vi "Driveshift.vi"(7 "GO BUTTON":bool, 10 "Shift down override":bool, 11 "Shift up override":bool) -> ()   [LabVIEW 2013]
uses:
  <vilib>/Rock Robotics/WPI/Solenoid/WPI_SolenoidValue.ctl
  Robot Global Data.vi
  <vilib>/Rock Robotics/WPI/Solenoid/WPI_SolenoidSetEnum.vi
panel:
  out "Solenoid Value":T1
  in  "Shift Speed":dbl=4.5
  in  "Value":bool
  in  "DOWN Shift Speed":dbl=1.0
  in  "UP Shift Speed":dbl=4.5
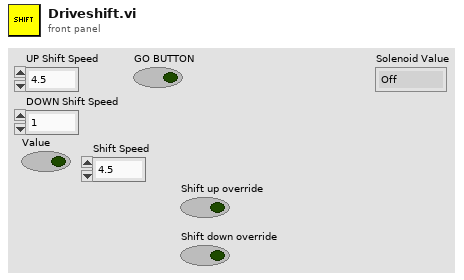
[diagram p1: front panel]
types:
  T1 = typedef "WPI_SolenoidValue.ctl" = enum16{"Off", "On", "Forward", "Reverse"}
  T2 = typedef "WPI_EncoderDevRef.ctl" = cluster{"DevStatus":errorcluster, "EncoderIndex":T3, "CounterIndex":T4, "DistancePerCount":dbl, "Decoding Type":T5}
  T3 = typedef "FPGA_EncoderIdx.ctl" = enum8{"Enc 0", "Enc 1", "Enc 2", "Enc 3", "Invalid"}
  T4 = typedef "FPGA_CounterCtrSystemIndex.ctl" = enum8{"Ctr 0", "Ctr 1", "Ctr 2", "Ctr 3", "Ctr 4", "Ctr 5", "Ctr 6", "Ctr 7", "Invalid"}
  T5 = typedef "WPI_EncoderType.ctl" = enum16{"1x", "2x", "4x"}
  T6 = typedef "WPI_SolenoidDevRef.ctl" = cluster{"DevStatus":errorcluster, "Solenoid Module":T7, "Forward Solenoid Channel":T8, "Reverse Solenoid Channel":T8}
  T7 = typedef "FPGA_TypedefSolenoidModule.ctl" = enum16{"Solenoid Module 1", "Solenoid Module 2"}
  T8 = typedef "WPI_SolenoidChannel.ctl" = enum8{"Solenoid 1", "Solenoid 2", "Solenoid 3", "Solenoid 4", "Solenoid 5", "Solenoid 6", "Solenoid 7", "Solenoid 8", "Invalid"}
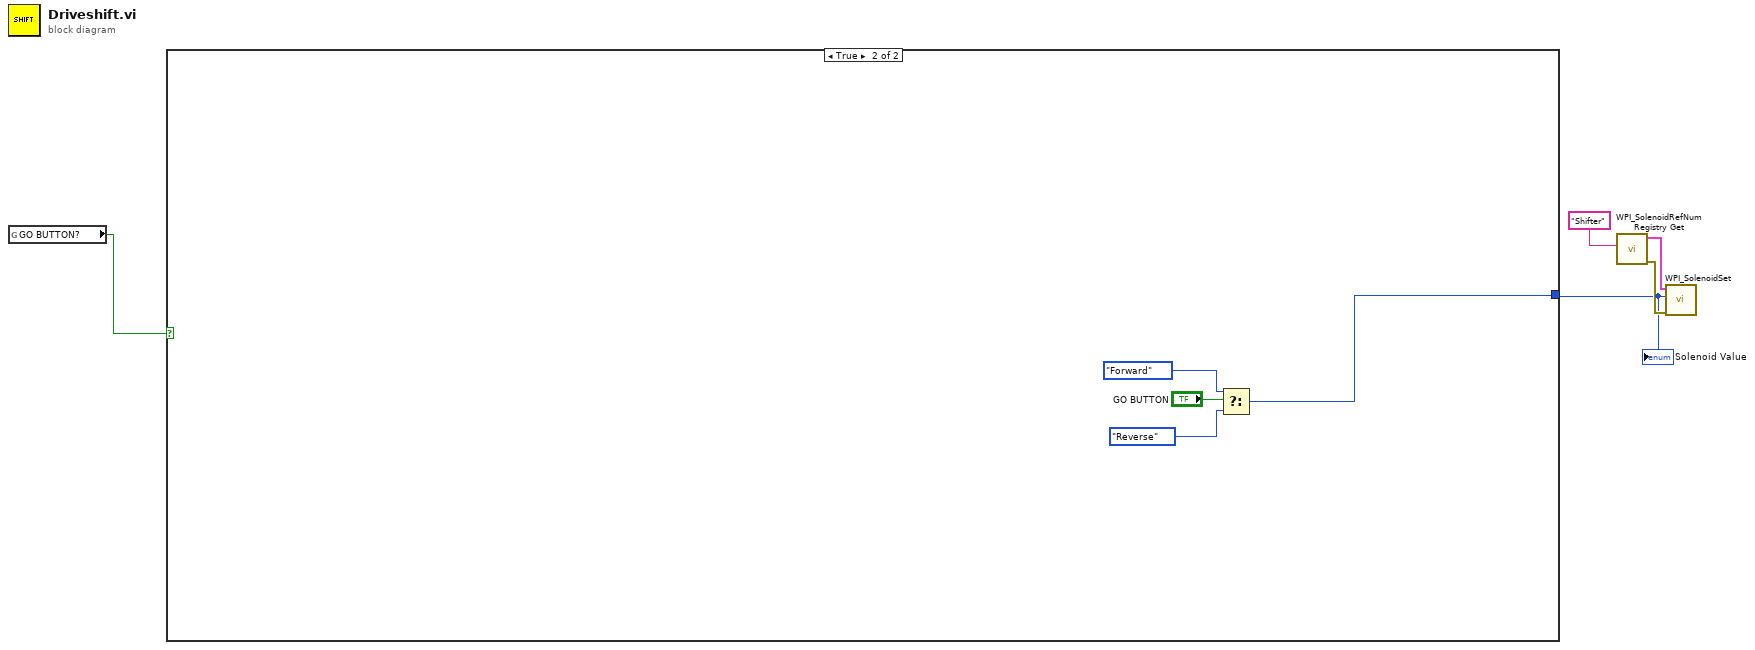
[diagram p0: block diagram]
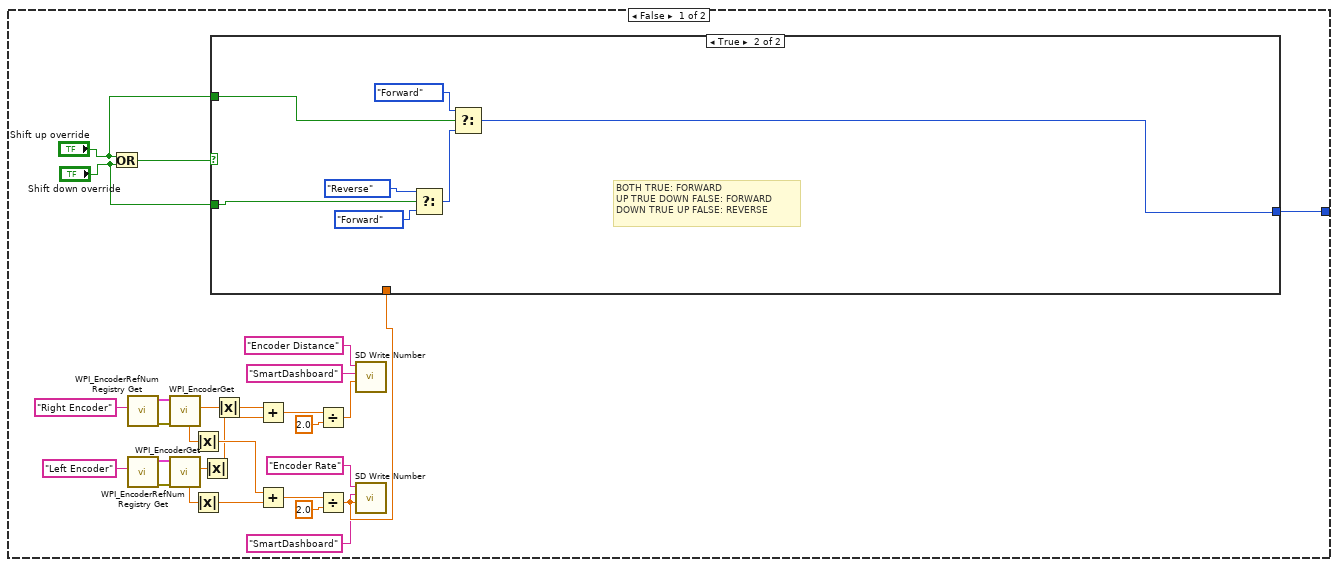
[diagram p2: hidden frame]
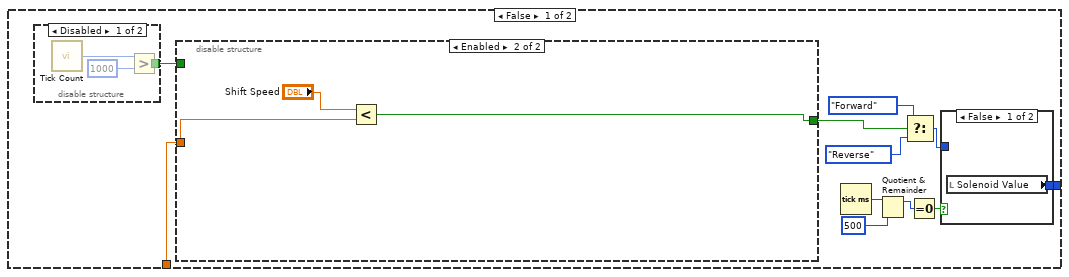
[diagram p3: hidden frame]
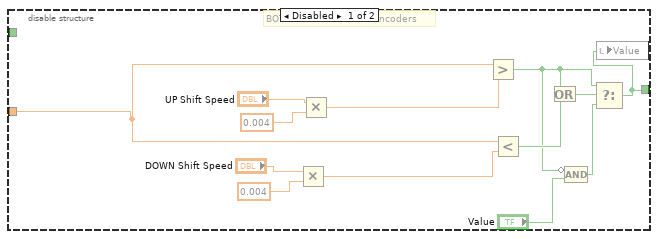
[diagram p6: hidden frame]
diagram:
  n1 = global read "Robot Global Data.vi" "GO BUTTON?"() -> (w1:bool)
  n2 = case shown="True" w1 {
    tunnel: [w6 w75] -> w3
    frame False {
      n3 = Or(x="Shift up override", y="Shift down override") -> (x .or. y?=w33:bool)
      n4 = call <vilib>:"WPI_EncoderRefNum Registry Get.vi"("refnum name"="Right Encoder") -> ("error out"=w22:errorcluster, "EncoderDevRef"=w23:T2)  [unwired: 9 in]
      n5 = call <vilib>:"WPI_EncoderRefNum Registry Get.vi"("refnum name"="Left Encoder") -> ("error out"=w25:errorcluster, "EncoderDevRef"=w24:T2)  [unwired: 9 in]
      n6 = call <vilib>:"WPI_EncoderGet.vi"("error in (no error)"=w22, "EncoderDevRef"=w23) -> ("Distance"=w13:dbl, "Rate"=w29:dbl)  [unwired: 4 in, 4 out]
      n7 = call <vilib>:"WPI_EncoderGet.vi"("error in (no error)"=w25, "EncoderDevRef"=w24) -> ("Distance"=w12:dbl, "Rate"=w30:dbl)  [unwired: 4 in, 4 out]
      n8 = Absolute Value(x=w29) -> (abs(x)=w10:dbl)
      n9 = Absolute Value(x=w30) -> (abs(x)=w9:dbl)
      n10 = Absolute Value(x=w12) -> (abs(x)=w8:dbl)
      n11 = Absolute Value(x=w13) -> (abs(x)=w7:dbl)
      n12 = Add(x=w7, y=w8) -> (x+y=w15:dbl)
      n13 = Add(x=w10, y=w9) -> (x+y=w27:dbl)
      n14 = Divide(x=w15, y=2.0) -> (x/y=w11:dbl)
      n15 = Divide(x=w27, y=2.0) -> (x/y=w20:dbl)
      n16 = case shown="True" w33 {
        tunnel: "Shift up override" -> [_ w72]
        tunnel: "Shift down override" -> [_ w70]
        tunnel: [w39 w67] -> w6
        tunnel: w20 -> [w41 _]
        frame False {
          n17 = disable-structure shown="Disabled" {
            disable-tunnel: [w47 _] -> w40
            frame Disabled {
              n18 = call "Tick Count"() -> ("Tick Count(mSec)"=w49:u32)
              n19 = Greater?(x=w49, y=u32 1000) -> (0:w47:bool)
            }
            frame Enabled {
            }
          }
          n20 = disable-structure shown="Enabled" {
            disable-tunnel: [w51 w63] -> w44
            disable-tunnel: w41 -> [w50 w64]
            disable-tunnel: w40 -> [_ _]
            frame Disabled {
              # "BOTH FALSE: examine encoders"
              n21 = Multiply(x="DOWN Shift Speed", y=0.004) -> (x*y=w52:dbl)
              n22 = Multiply(x="UP Shift Speed", y=0.004) -> (x*y=w55:dbl)
              n23 = Greater?(x=w50, y=w55) -> (0:w60:bool)
              n24 = Less?(x=w50, y=w52) -> (x < y?=w61:bool)
              n25 = Or(x=w60, y=w61) -> (x .or. y?=w62:bool)
              n26 = Compound Arithmetic op=AND(invert w60, "Value") -> (w59:bool)
              n27 = Select(t=w60, s=w62, f=w59) -> (s? t:f=w51:bool)
              n28 = local write "Value"(w51) -> ()
            }
            frame Enabled {
              n29 = Less?(x="Shift Speed", y=w64) -> (x < y?=w63:bool)
            }
          }
          n30 = Tick Count (ms)() -> (millisecond timer value=w38:u32)
          n31 = Quotient & Remainder(x=w38, y=u32 500) -> (x-y*floor(x/y)=w35:u32)  [unwired: 1 out]
          n32 = Select(t=WPI_SolenoidValue."Forward" ("Value"), s=w44, f=WPI_SolenoidValue."Reverse" ("Value")) -> (s? t:f=w34:T1)
          n33 = Equal To 0?(x=w35) -> (x = 0?=w36:bool)
          n34 = case shown="False" w36 {
            tunnel: w34 -> [_ w46]
            tunnel: [w45 w46] -> w39
            frame False {
              n35 = local read "Solenoid Value"() -> (w45:T1)
            }
            frame True {
            }
          }
        }
        frame True {
          # "BOTH TRUE: FORWARD \nUP TRUE DOWN FALSE: FORWARD\nDOWN TRUE UP FALSE: REVERSE"
          n36 = Select(t=WPI_SolenoidValue."Reverse" ("f"), s=w70, f=WPI_SolenoidValue."Forward") -> (s? t:f=w66:T1)
          n37 = Select(t=WPI_SolenoidValue."Forward" ("Value"), s=w72, f=w66) -> (s? t:f=w67:T1)
        }
      }
      n38 = call <vilib>:"SD Write Number.vi"("Numeric"=w11, "Table Prefix"="SmartDashboard", "Name"="Encoder Distance") -> ()  [unwired: 7 in, 2 out]
      n39 = call <vilib>:"SD Write Number.vi"("Numeric"=w20, "Table Prefix"="SmartDashboard", "Name"="Encoder Rate") -> ()  [unwired: 7 in, 2 out]
    }
    frame True {
      n40 = Select(t=WPI_SolenoidValue."Forward" ("f"), s="GO BUTTON", f=WPI_SolenoidValue."Reverse") -> (s? t:f=w75:T1)
    }
  }
  "Solenoid Value" <- w3
  n41 = call <vilib>:"WPI_SolenoidRefNum Registry Get.vi"("refnum name"="Shifter") -> ("error out"=w5:errorcluster, "SolenoidDevRef"=w4:T6)  [unwired: 9 in]
  n42 = call-poly <vilib>:"WPI_SolenoidSet.vi"("error in (no error)"=w5, "Value"=w3, "SolenoidDevRef"=w4) -> ()  [unwired: 7 in, 2 out]
